vi "SetSprites.vi"(8 "error in (no error)":errorcluster, 10 "Array":refnum<class "RT_Sprite.lvclass">[](array[class]), 11 "MainMenu in":refnum<class "Game.lvclass">) -> (0 "error out":errorcluster, 3 "MainMenu out":refnum<class "Game.lvclass">)   [LabVIEW 2019, in "RT_Game.lvlib" / "Game.lvclass"]
uses:
  Game.lvclass
  RT_Sprite/RT_Sprite.lvclass
  Game.lvclass/Game.ctl
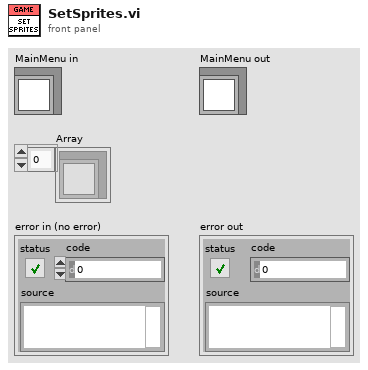
[diagram p1: front panel]
types:
  T1 = cluster{"Array[0]":refnum<class "RT_Sprite.lvclass">, "Array[1]":refnum<class "RT_Sprite.lvclass">, "Array[2]":refnum<class "RT_Sprite.lvclass">}
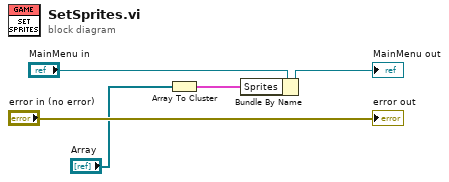
[diagram p0: block diagram]
diagram:
  n1 = Array To Cluster(array="Array") -> (cluster=w1:T1)
  n2 = Bundle By Name(cluster="MainMenu in", "Sprites"=w1) -> (→"MainMenu out":refnum<class "Game.lvclass">)
  "error out" <- "error in (no error)"
